vi "VALEW_Rename DAQmx Devices.vi"(0 "cDAQ Name":string, 11 "Error In":errorcluster) -> (15 "Error Out":errorcluster)   [LabVIEW 2016, in "Centauro.lvlib"]
uses:
  Projects/Centauro.lvlib
  <vilib>/nisyscfg/Initialize (Control).vi
  <vilib>/nisyscfg/Find Hardware.vi
  <vilib>/nisyscfg/Close (Filter).vi
  <vilib>/nisyscfg/Close (Hardware).vi
  <vilib>/nisyscfg/Close (System).vi
  <vilib>/nisyscfg/nisyscfg.lvlib
  <resource>/objmgr/nisysapi.rc
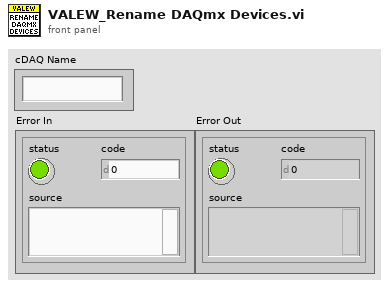
[diagram p1: front panel]
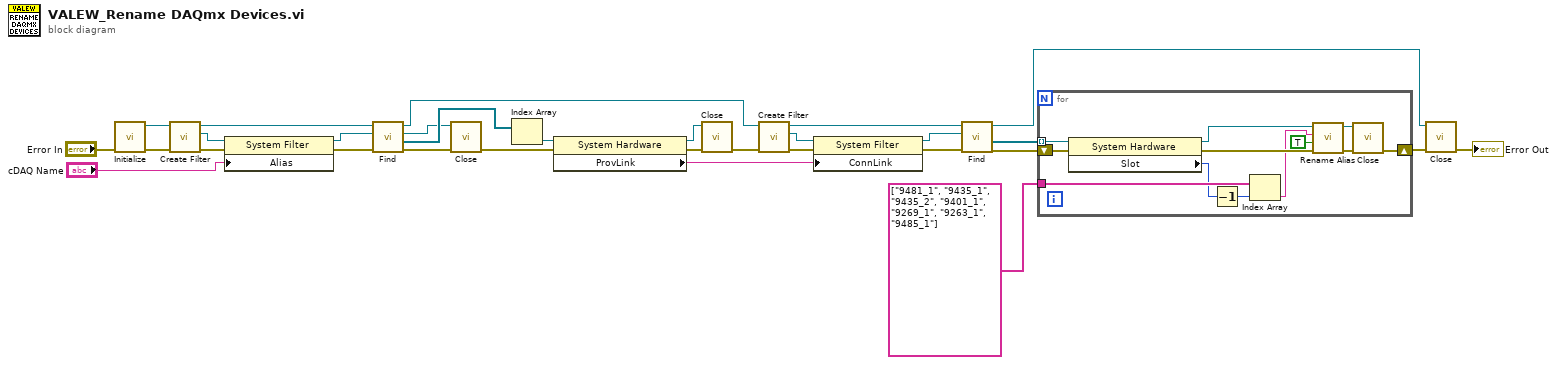
[diagram p0: block diagram]
diagram:
  n1 = call-poly <vilib>:"Initialize.vi"("error in (no error)"="Error In") -> ("error out"=w29:errorcluster, "Session out"=w30:refnum<k21>)  [unwired: 8 in, 1 out]
  n2 = call <vilib>:"Create Filter.vi"("error in (no error)"=w29, "Session in"=w30) -> ("error out"=w27:errorcluster, "Filter out"=w28:refnum<k20>, "Session out"=w26:refnum<k21>)  [unwired: 7 in]
  n3 = property class="System Filter"(reference=w28, error in=w27, "Alias"="cDAQ Name") -> (reference out=w23:refnum<k20>, error out=w25:errorcluster)
  n4 = call-poly <vilib>:"Find.vi"("error in (no error)"=w25, "Filter in"=w23, "Session in"=w26) -> ("error out"=w12:errorcluster, "Resources out"=w20:refnum<k20>[], "Filter out"=w13:refnum<k20>, "Session out"=w10:refnum<k21>)  [unwired: 5 in]
  n5 = call-poly <vilib>:"Close.vi"("error in (no error)"=w12, "Filter in"=w13) -> ("error out"=w11:errorcluster)  [unwired: 9 in]
  n6 = Index Array(array=w20) -> (element=w19:refnum<k20>)  [unwired: 1 in]
  n7 = property class="System Hardware"(reference=w19, error in=w11) -> (reference out=w9:refnum<k20>, error out=w8:errorcluster, "ProvLink"=w6:string)
  n8 = call-poly <vilib>:"Close.vi"("error in (no error)"=w8, "Resource in"=w9) -> ("error out"=w7:errorcluster)  [unwired: 9 in]
  n9 = call <vilib>:"Create Filter.vi"("error in (no error)"=w7, "Session in"=w10) -> ("error out"=w15:errorcluster, "Filter out"=w14:refnum<k20>, "Session out"=w16:refnum<k21>)  [unwired: 7 in]
  n10 = property class="System Filter"(reference=w14, error in=w15, "ConnLink"=w6) -> (reference out=w18:refnum<k20>, error out=w17:errorcluster)
  n11 = call-poly <vilib>:"Find.vi"("error in (no error)"=w17, "Filter in"=w18, "Session in"=w16) -> ("error out"=w3:errorcluster, "Resources out"=w4:refnum<k20>[], "Session out"=w2:refnum<k21>)  [unwired: 5 in, 1 out]
  n12 = for {
    tunnel: string[] ["9481_1", "9435_1", "9435_2", "9401_1", "9269_1", "9263_1", "9485_1"] -> [w40]
    tunnel: w4 -> [w42] mode=indexing
    shift-right: [w36] -> w1
    shift-left: w3 -> [w41]
    n13 = property class="System Hardware"(reference=w42, error in=w41) -> (reference out=w34:refnum<k20>, error out=w37:errorcluster, "Slot"=w31:i32)
    n14 = Decrement(x=w31) -> (x-1=w32:i32)
    n15 = Index Array(array=w40, index=w32) -> (element=w35:string)
    n16 = call <vilib>:"Rename Alias.vi"("error in (no error)"=w37, "Overwrite Conflict (F)"=TRUE ("overwrite (F)"), "New Name"=w35, "Resource in"=w34) -> ("error out"=w38:errorcluster, "Resource out"=w33:refnum<k20>)  [unwired: 4 in, 2 out]
    n17 = call-poly <vilib>:"Close.vi"("error in (no error)"=w38, "Resource in"=w33) -> ("error out"=w36:errorcluster)  [unwired: 9 in]
  }
  n18 = call-poly <vilib>:"Close.vi"("error in (no error)"=w1, "Session in"=w2) -> ("error out"=→"Error Out":errorcluster)  [unwired: 9 in]
